vi "dispense example.vi"() -> ()   [LabVIEW 2016]
uses:
  Classes/Controller/Dispenser/Ultimus V2 Folder/Ultimus V2.lvclass
panel:
  in  "stop":bool
  in  "change status":bool=TRUE
  in  "Array":dbl[](array[numeric])=[0.0, 0.0]
  in  "Start":bool=TRUE
  in  "Delay Time (s)":dbl=1.0
  in  "Pressure (psi)":i16
  in  "Vacuum Setting (0000)":i64 min=0 max=1000 step=1 format="%04.0f"
  # "This vi will control the dispenser to dispense ... seconds"
  # "0123 -> 01.23 kPa ( Max 4.45kPa )"
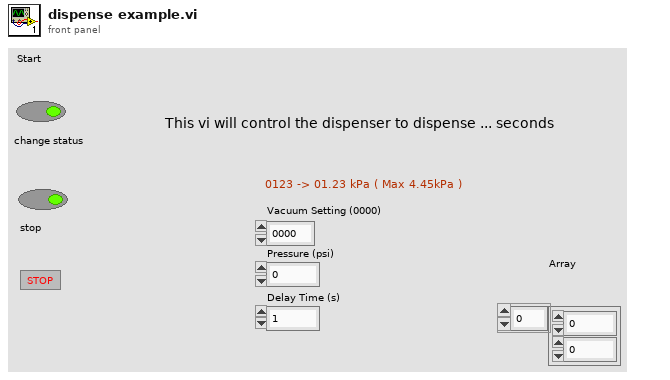
[diagram p1: front panel]
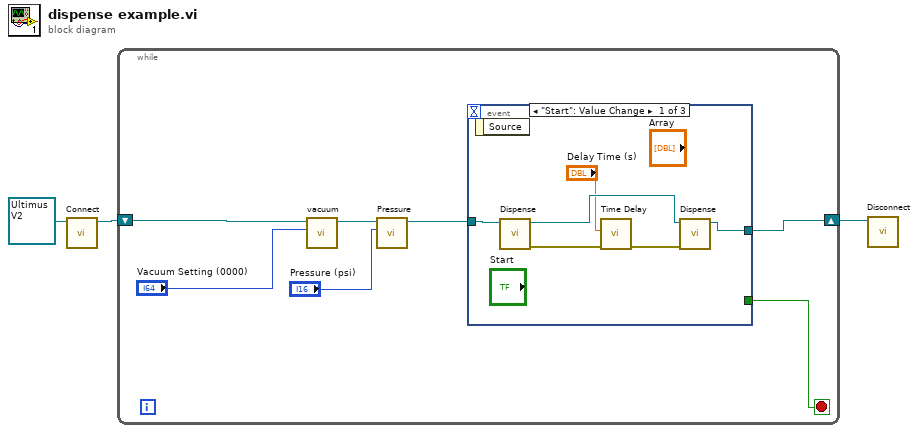
[diagram p0: block diagram]
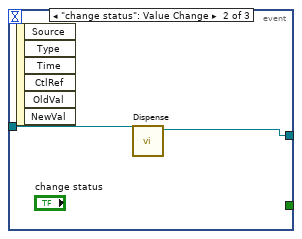
[diagram p2: hidden frame]
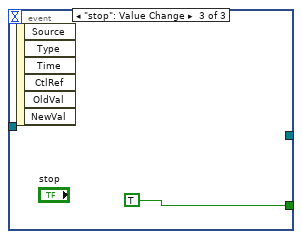
[diagram p3: hidden frame]
diagram:
  n1 = call-dynamic "Connect.vi"("Ultimus V in"=refnum<class "Ultimus V2.lvclass"> refnum ("Ultimus V2.lvclass")) -> ("Ultimus V out"=w2:refnum<class "Ultimus V2.lvclass">)  [unwired: 9 in, 1 out]
  n2 = while {
    shift-right: [w5] -> w1
    shift-left: w2 -> [w10]
    stop <- w4 stop-if-true
    n3 = call "vacuum.vi"("Vacuum Setting (0000)"="Vacuum Setting (0000)", "Ultimus V in"=w10) -> ("Ultimus V out"=w9:refnum<class "Ultimus V2.lvclass">)  [unwired: 8 in, 1 out]
    n4 = call-dynamic "Pressure.vi"("Pressure"="Pressure (psi)", "Ultimus V in"=w9) -> ("Ultimus V out"=w8:refnum<class "Ultimus V2.lvclass">)  [unwired: 8 in, 1 out]
    n5 = event shown="[0] \"Start\": Value Change" {
      selector: _ -> [_ _ _]
      dyn-events: _ -> [_ _ _]
      timeout: _ -> [_ _ _]
      tunnel: w8 -> [w12 w18 _]
      tunnel: [w11 w17 _] -> w5
      tunnel: [_ _ TRUE] -> w4
      event "Start": Value Change {
        n6 = event-data() -> ()  [unwired: 1 in, 1 out]
        n7 = call-dynamic "Dispense.vi"("Ultimus V in"=w12) -> ("error out"=w16:errorcluster, "Ultimus V out"=w14:refnum<class "Ultimus V2.lvclass">)  [unwired: 9 in]
        n8 = call "Time Delay"("error in (no error)"=w16, "Delay Time (s)"="Delay Time (s)") -> ("error out"=w15:errorcluster)  [unwired: 9 in]
        n9 = call-dynamic "Dispense.vi"("error in (no error)"=w15, "Ultimus V in"=w14) -> ("Ultimus V out"=w11:refnum<class "Ultimus V2.lvclass">)  [unwired: 8 in, 1 out]
      }
      event "change status": Value Change {
        n10 = event-data() -> ()  [unwired: 1 in, 6 out]
        n11 = call-dynamic "Dispense.vi"("Ultimus V in"=w18) -> ("Ultimus V out"=w17:refnum<class "Ultimus V2.lvclass">)  [unwired: 9 in, 1 out]
      }
      event "stop": Value Change {
        n12 = event-data() -> ()  [unwired: 1 in, 6 out]
      }
    }
  }
  n13 = call-dynamic "Disconnect.vi"("Ultimus V in"=w1) -> ()  [unwired: 9 in, 1 out]
